vi "TDMS_FileLocationErrorMessage.vi"(10 "fileLocation":path, 11 "errorIn":errorcluster) -> (0 "errorCode":i32, 1 "buttonStatus":bool)   [LabVIEW 2021]
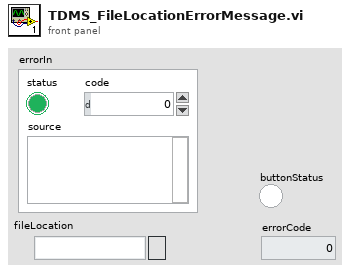
[diagram p1: front panel]
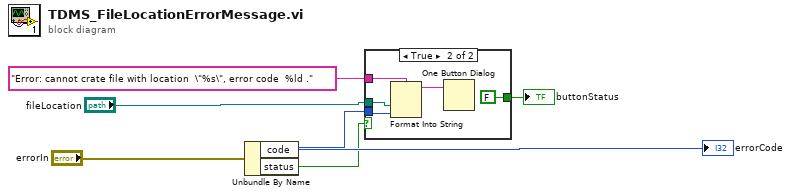
[diagram p0: block diagram]
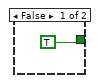
[diagram p2: hidden frame]
diagram:
  n1 = Unbundle By Name("errorIn") -> ("code"=w6:i32, "status"=w3:bool)
  "errorCode" <- w6
  n2 = case shown="True" w3 {
    tunnel: w6 -> [_ w10]
    tunnel: "Error: cannot crate file with location  \"%s\", error code  %ld ." ("format string") -> [_ w11]
    tunnel: "fileLocation" -> [_ w9]
    tunnel: [TRUE FALSE] -> w1
    frame False {
    }
    frame True {
      n3 = Format Into String(format string=w11, w9, w10) -> (resulting string=w12:string)  [unwired: 2 in, 1 out]
      n4 = One Button Dialog(message=w12) -> ()  [unwired: 1 in, 1 out]
    }
  }
  "buttonStatus" <- w1
